vi "Theme Entry Enum To String.vi"(11 "Root Theme Entry":T1) -> (3 "Root Theme Entry String":string)   [LabVIEW 2021, in "Appearance Actor.lvlib" / "Generic Theme.lvclass"]
uses:
  Generic Theme.lvclass
  Typedefs/Theme Entry--enum.ctl
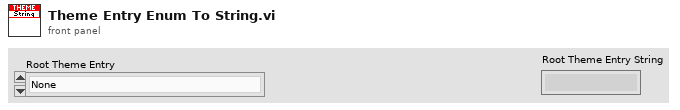
[diagram p1: front panel]
types:
  T1 = typedef "Appearance Actor.lvlib/Generic Theme.lvclass/Theme Entry--enum.ctl" = enum16{"None", "TitleBar.Pane.Color", "TitleBar.Splitter.FillColor", "TitleBar.Splitter.OutlineColor", "TitleBar.Title.Font.Color", "TitleBar.Title.Font.Family", "TitleBar.Title.Font.Size", "TitleBar.Title.Font.Style"}
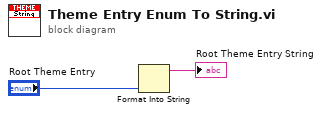
[diagram p0: block diagram]
diagram:
  n1 = Format Into String("Root Theme Entry") -> (resulting string=→"Root Theme Entry String":string)  [unwired: 3 in, 1 out]
